vi "AddressRef.vi"(7 "Init":bool, 9 "prrty in":refnum<vi>, 10 "add_type in":refnum<vi>, 11 "add_dst in":refnum<vi>) -> (1 "prrty out":refnum<vi>, 2 "add_type out":refnum<vi>, 3 "add_dst out":refnum<vi>)   [LabVIEW 2017]
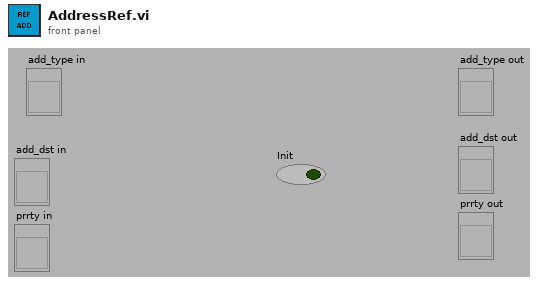
[diagram p1: front panel]
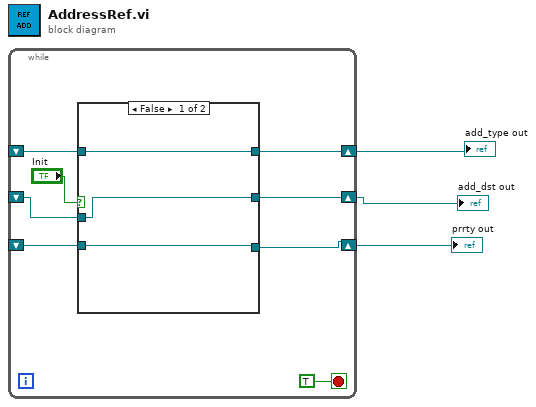
[diagram p0: block diagram]
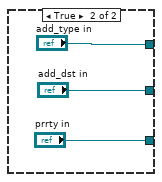
[diagram p2: hidden frame]
diagram:
  n1 = while {
    shift-right: [w10] -> w3
    shift-left: _ -> [w8]
    shift-right: [w7] -> w2
    shift-left: _ -> [w5]
    shift-right: [w6] -> w1
    shift-left: _ -> [w4]
    stop <- TRUE stop-if-true
    n2 = case shown="False" "Init" {
      tunnel: [w14 "add_type in"] -> w10
      tunnel: w8 -> [w14 _]
      tunnel: [w13 "add_dst in"] -> w7
      tunnel: [w12 "prrty in"] -> w6
      tunnel: w5 -> [w13 _]
      tunnel: w4 -> [w12 _]
      frame False {
      }
      frame True {
      }
    }
  }
  "add_type out" <- w3
  "add_dst out" <- w2
  "prrty out" <- w1
